vi "Discovery Management Core.vi"(11 "CIFPluginManager in":refnum<class "CIFPluginManager.lvclass">) -> (0 "error out":errorcluster)   [LabVIEW 2021, in "CIFPluginManager.lvclass"]
uses:
  CIFPluginManager.lvclass
  typedef/Discover Command.ctl
  CIFPluginManager.lvclass/CIFPluginManager.ctl
  CIFUtilities/CIFLogs/CIFLogs.lvlib
  gRPC/CIF_Manager_Client_Wrapper/CIFManagerClientWrapper.lvlib
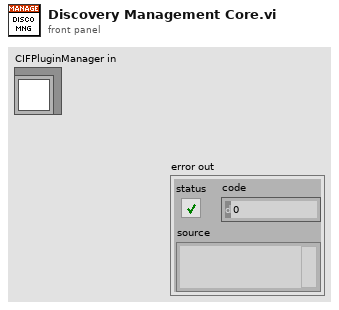
[diagram p1: front panel]
types:
  T1 = typedef "CIFPluginManager.lvclass/Discover Command.ctl" = cluster{"Loader Name":string, "Update Metadata":bool}
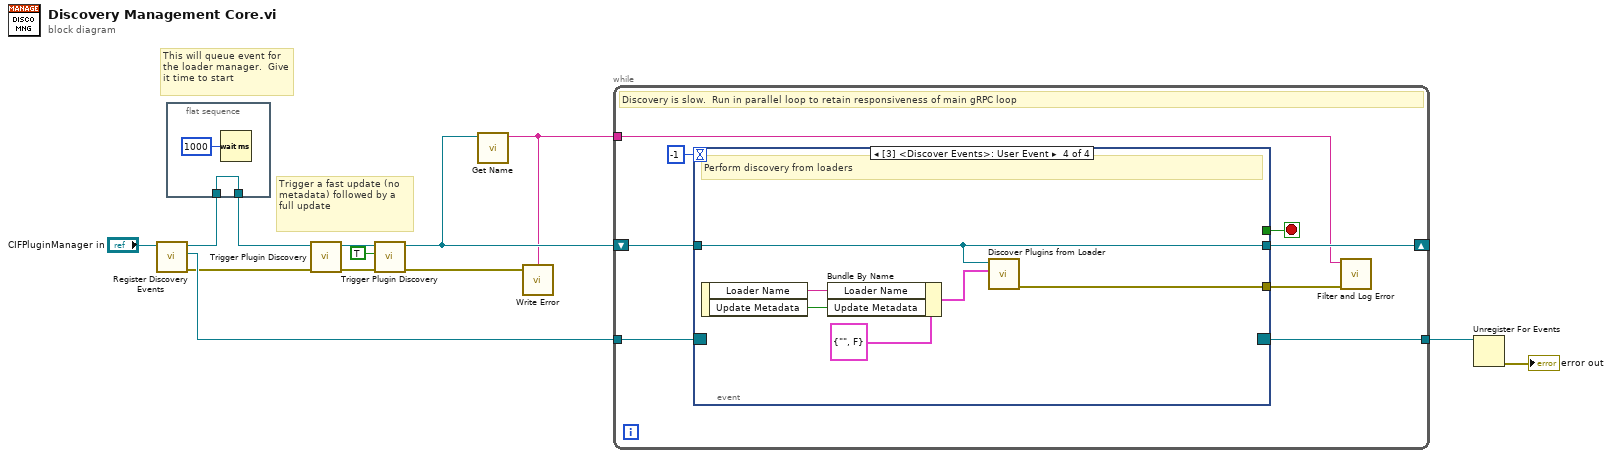
[diagram p0: block diagram]
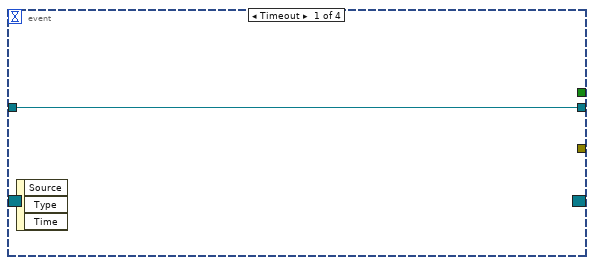
[diagram p2: hidden frame]
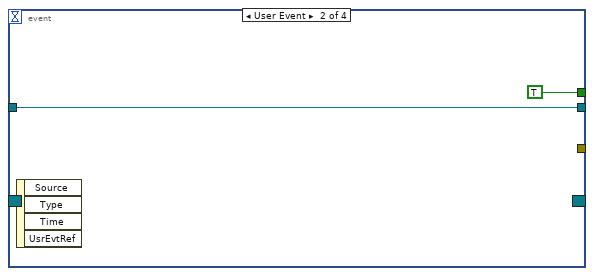
[diagram p3: hidden frame]
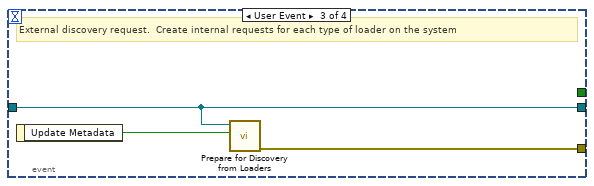
[diagram p4: hidden frame]
diagram:
  # "This will queue event for the loader manager.  Give it time to start"
  # "Trigger a fast update (no metadata) followed by a full update"
  n1 = call "Register Discovery Events.vi"("CIFPluginManager in"="CIFPluginManager in") -> ("error out"=w9:errorcluster, "Event Registration Refnum"=w11:refnum<event-registration>, "CIFPluginManager out"=w2:refnum<class "CIFPluginManager.lvclass">)  [unwired: 8 in]
  n2 = flat-sequence {
    tunnel: [w15] -> w1
    tunnel: w2 -> [w15]
    frame #0 {
      n3 = Wait (ms)(milliseconds to wait=u32 1000) -> ()  [unwired: 1 out]
    }
  }
  n4 = call "Trigger Plugin Discovery.vi"("error in (no error)"=w9, "CIFPluginManager in"=w1) -> ("error out"=w7:errorcluster, "CIFPluginManager out"=w8:refnum<class "CIFPluginManager.lvclass">)  [unwired: 8 in]
  n5 = call "Trigger Plugin Discovery.vi"("error in (no error)"=w7, "Update Metadata"=TRUE, "CIFPluginManager in"=w8) -> ("error out"=w6:errorcluster, "CIFPluginManager out"=w4:refnum<class "CIFPluginManager.lvclass">)  [unwired: 7 in]
  n6 = call "Get Name.vi"("CIFPluginManager in"=w4) -> ("Name"=w3:string)  [unwired: 10 in]
  n7 = call "Write Error.vi"("error in (no error)"=w6, "Plugin Name"=w3) -> ()  [unwired: 2 in, 1 out]
  n8 = while {
    tunnel: w11 -> [w17]
    shift-right: [w21] -> _
    shift-left: w4 -> [w23]
    tunnel: [w19] -> w12
    tunnel: w3 -> [w16]
    stop <- w20 stop-if-true
    # "Discovery is slow.  Run in parallel loop to retain responsiveness of main gRPC loop"
    n9 = event shown="[3] <Discover Events>: User Event" {
      selector: w17 -> [_ _ _ _]
      dyn-events: [_ _ _ _] -> w19
      timeout: -1 -> [_ _ _ _]
      tunnel: w23 -> [w24 w25 w28 w34]
      tunnel: [w24 w25 w28 w34] -> w21
      tunnel: [_ TRUE _ _] -> w20
      tunnel: [_ _ w27 w35] -> w18
      event Timeout {
        n10 = event-data() -> ()  [unwired: 1 in, 3 out]
      }
      event User Event {
        n11 = event-data() -> ()  [unwired: 1 in, 4 out]
      }
      event User Event {
        # "External discovery request.  Create internal requests for each type of loader on the system"
        n12 = event-data() -> ("Update Metadata"=w29:bool)  [unwired: 1 in]
        n13 = call "Prepare for Discovery from Loaders.vi"("Update Metadata"=w29, "CIFPluginManager in"=w28) -> ("error out"=w27:errorcluster)  [unwired: 9 in]
      }
      event User Event {
        # "Perform discovery from loaders"
        n14 = event-data() -> ("Loader Name"=w32:string, "Update Metadata"=w31:bool)  [unwired: 1 in]
        n15 = Bundle By Name(cluster=T1 {"Loader Name"="", "Update Metadata"=FALSE} ("Discovery Command"), "Loader Name"=w32, "Update Metadata"=w31) -> (w30:T1)
        n16 = call "Discover Plugins from Loader.vi"("Discovery Command"=w30, "CIFPluginManager in"=w34) -> ("error out"=w35:errorcluster)  [unwired: 9 in]
      }
    }
    n17 = call "Filter and Log Error.vi"("error In"=w18, "Name"=w16) -> ()  [unwired: 10 in]
  }
  n18 = Unregister For Events(event registration refnum=w12) -> (error out=→"error out":errorcluster)  [unwired: 1 in]
